vi "Value setter.vi"(2 "Array":i16[](array[numeric]), 3 "Enum":enum16{"FWD", "CL", "CT", "Ar", "O2", "Timer"}(ring), 4 "value":i32) -> (0 "output array":i16[](array[numeric]), 1 "value":i16)   [LabVIEW 2023]
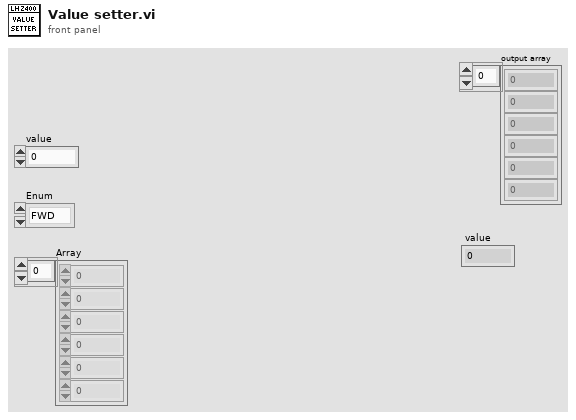
[diagram p1: front panel]
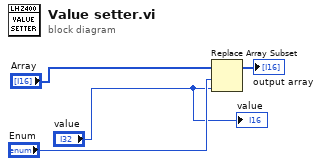
[diagram p0: block diagram]
diagram:
  n1 = Replace Array Subset(array="Array", new element="value", index="Enum") -> (→"output array":i16[])
  "value" <- "value"
